vi "Lab Panel V5.31.vi"() -> ()   [LabVIEW 2017] (continued)
                        n3241 = Unbundle By Name(w5920) -> ("1 (TL) cal"=w5915:dbl, "1 (TN) cal"=w5914:dbl, "2 (TL) cal"=w5913:dbl, "2 (TN) cal"=w5912:dbl)  [unwired: 6 out]
                        n3242 = local write "TEMP LA03"(w5909) -> ()
                        n3243 = Multiply(x=w5908, y=w5915) -> (x*y=w5901:dbl)
                        n3244 = Multiply(x=w5907, y=w5914) -> (x*y=w5900:dbl)
                        n3245 = Multiply(x=w5906, y=w5913) -> (x*y=w5897:dbl)
                        n3246 = Multiply(x=w5905, y=w5912) -> (x*y=w5896:dbl)
                        n3247 = case shown="True" w5892 {
                          tunnel: w5897 -> [w5922 w5927]
                          tunnel: w5902 -> [_ w5925]
                          tunnel: [w5922 w5926] -> w5895
                          tunnel: w5896 -> [w5921 w5924]
                          tunnel: [w5921 w5923] -> w5894
                          frame False {
                          }
                          frame True {
                            n3248 = Multiply(x=w5925, y=w5924) -> (x*y=w5923:dbl)
                            n3249 = Multiply(x=w5925, y=w5927) -> (x*y=w5926:dbl)
                          }
                        }
                        n3250 = case shown="True" w5893 {
                          tunnel: w5901 -> [w5929 w5934]
                          tunnel: w5902 -> [_ w5932]
                          tunnel: [w5929 w5933] -> w5899
                          tunnel: w5900 -> [w5928 w5931]
                          tunnel: [w5928 w5930] -> w5898
                          frame False {
                          }
                          frame True {
                            n3251 = Multiply(x=w5932, y=w5931) -> (x*y=w5930:dbl)
                            n3252 = Multiply(x=w5932, y=w5934) -> (x*y=w5933:dbl)
                          }
                        }
                        n3253 = local read "SIG LAB03-2"() -> (w5917:T2)
                        n3254 = local read "SIG LAB03-1"() -> (w5919:T2)
                        n3255 = Bundle By Name(cluster=w5917, "Tmp Live"=w5895, "Tmp Neut"=w5894) -> (w5916:T2)
                        n3256 = Bundle By Name(cluster=w5919, "Tmp Live"=w5899, "Tmp Neut"=w5898) -> (w5918:T2)
                        n3257 = local write "SIG LAB03-2"(w5916) -> ()
                        n3258 = local write "SIG LAB03-1"(w5918) -> ()
                      }
                      frame #4 {
                        n3259 = case shown="False" w5949 {
                          tunnel: [w5980 w5981] -> w5965
                          tunnel: w5948 -> [_ w5981]
                          frame False {
                            n3260 = local read "CAL LAB04"() -> (w5980:T15)
                          }
                          frame True {
                          }
                        }
                        n3261 = local read "LAB04 TEMP"() -> (w5955:T13)
                        n3262 = local read "TEMP LA04"() -> (w5956:T10)
                        n3263 = call "sub vi - temperature delay v4.vi"("2-run"=w5937, "1-run"=w5938, "temp values IN"=w5956, "temp signals"=w5955) -> ("T2-N"=w5950:dbl, "T2-L"=w5951:dbl, "T1-N"=w5952:dbl, "T1-L"=w5953:dbl, "temp values OUT"=w5954:T47)  [unwired: 3 in]
                        n3264 = Unbundle By Name(w5965) -> ("1 (TL) cal"=w5960:dbl, "1 (TN) cal"=w5959:dbl, "2 (TL) cal"=w5958:dbl, "2 (TN) cal"=w5957:dbl)  [unwired: 6 out]
                        n3265 = local write "TEMP LA04"(w5954) -> ()
                        n3266 = Multiply(x=w5953, y=w5960) -> (x*y=w5946:dbl)
                        n3267 = Multiply(x=w5952, y=w5959) -> (x*y=w5945:dbl)
                        n3268 = Multiply(x=w5951, y=w5958) -> (x*y=w5942:dbl)
                        n3269 = Multiply(x=w5950, y=w5957) -> (x*y=w5941:dbl)
                        n3270 = case shown="True" w5937 {
                          tunnel: w5942 -> [w5967 w5972]
                          tunnel: w5947 -> [_ w5970]
                          tunnel: [w5967 w5971] -> w5940
                          tunnel: w5941 -> [w5966 w5969]
                          tunnel: [w5966 w5968] -> w5939
                          frame False {
                          }
                          frame True {
                            n3271 = Multiply(x=w5970, y=w5969) -> (x*y=w5968:dbl)
                            n3272 = Multiply(x=w5970, y=w5972) -> (x*y=w5971:dbl)
                          }
                        }
                        n3273 = case shown="True" w5938 {
                          tunnel: w5946 -> [w5974 w5979]
                          tunnel: w5947 -> [_ w5977]
                          tunnel: [w5974 w5978] -> w5944
                          tunnel: w5945 -> [w5973 w5976]
                          tunnel: [w5973 w5975] -> w5943
                          frame False {
                          }
                          frame True {
                            n3274 = Multiply(x=w5977, y=w5976) -> (x*y=w5975:dbl)
                            n3275 = Multiply(x=w5977, y=w5979) -> (x*y=w5978:dbl)
                          }
                        }
                        n3276 = local read "SIG LAB04-2"() -> (w5962:T2)
                        n3277 = local read "SIG LAB04-1"() -> (w5964:T2)
                        n3278 = Bundle By Name(cluster=w5962, "Tmp Live"=w5940, "Tmp Neut"=w5939) -> (w5961:T2)
                        n3279 = Bundle By Name(cluster=w5964, "Tmp Live"=w5944, "Tmp Neut"=w5943) -> (w5963:T2)
                        n3280 = local write "SIG LAB04-2"(w5961) -> ()
                        n3281 = local write "SIG LAB04-1"(w5963) -> ()
                      }
                      frame #5 {
                        n3282 = case shown="False" w5994 {
                          tunnel: [w6025 w6026] -> w6010
                          tunnel: w5993 -> [_ w6026]
                          frame False {
                            n3283 = local read "CAL LAB05"() -> (w6025:T15)
                          }
                          frame True {
                          }
                        }
                        n3284 = local read "LAB05 TEMP"() -> (w6000:T13)
                        n3285 = local read "TEMP LA05"() -> (w6001:T10)
                        n3286 = call "sub vi - temperature delay v4.vi"("2-run"=w5982, "1-run"=w5983, "temp values IN"=w6001, "temp signals"=w6000) -> ("T2-N"=w5996:dbl, "T2-L"=w5997:dbl, "T1-N"=w5998:dbl, "T1-L"=w5999:dbl, "temp values OUT"=w5995:T47)  [unwired: 3 in]
                        n3287 = local write "TEMP LA05"(w5995) -> ()
                        n3288 = Unbundle By Name(w6010) -> ("1 (TL) cal"=w6002:dbl, "1 (TN) cal"=w6005:dbl, "2 (TL) cal"=w6004:dbl, "2 (TN) cal"=w6003:dbl)  [unwired: 6 out]
                        n3289 = Multiply(x=w5999, y=w6002) -> (x*y=w5991:dbl)
                        n3290 = Multiply(x=w5998, y=w6005) -> (x*y=w5990:dbl)
                        n3291 = Multiply(x=w5997, y=w6004) -> (x*y=w5987:dbl)
                        n3292 = Multiply(x=w5996, y=w6003) -> (x*y=w5986:dbl)
                        n3293 = case shown="True" w5982 {
                          tunnel: w5987 -> [w6012 w6017]
                          tunnel: w5992 -> [_ w6015]
                          tunnel: [w6012 w6016] -> w5985
                          tunnel: w5986 -> [w6011 w6014]
                          tunnel: [w6011 w6013] -> w5984
                          frame False {
                          }
                          frame True {
                            n3294 = Multiply(x=w6015, y=w6014) -> (x*y=w6013:dbl)
                            n3295 = Multiply(x=w6015, y=w6017) -> (x*y=w6016:dbl)
                          }
                        }
                        n3296 = case shown="True" w5983 {
                          tunnel: w5991 -> [w6019 w6024]
                          tunnel: w5992 -> [_ w6022]
                          tunnel: [w6019 w6023] -> w5989
                          tunnel: w5990 -> [w6018 w6021]
                          tunnel: [w6018 w6020] -> w5988
                          frame False {
                          }
                          frame True {
                            n3297 = Multiply(x=w6022, y=w6021) -> (x*y=w6020:dbl)
                            n3298 = Multiply(x=w6022, y=w6024) -> (x*y=w6023:dbl)
                          }
                        }
                        n3299 = local read "SIG LAB05-1"() -> (w6009:T2)
                        n3300 = Bundle By Name(cluster=w6009, "Tmp Live"=w5989, "Tmp Neut"=w5988) -> (w6008:T2)
                        n3301 = local read "SIG LAB05-2"() -> (w6007:T2)
                        n3302 = Bundle By Name(cluster=w6007, "Tmp Live"=w5985, "Tmp Neut"=w5984) -> (w6006:T2)
                        n3303 = local write "SIG LAB05-1"(w6008) -> ()
                        n3304 = local write "SIG LAB05-2"(w6006) -> ()
                      }
                      frame #6 {
                        w6127 = 150.0
                        # "check for thermocouple error, output >150 deg??"
                        n3305 = local read "SIG LAB01-2"() -> (w6136:T2)
                        n3306 = local read "SIG LAB01-1"() -> (w6137:T2)
                        n3307 = local read "SIG LAB04-1"() -> (w6130:T2)
                        n3308 = local read "SIG LAB04-2"() -> (w6131:T2)
                        n3309 = Unbundle By Name(w6137) -> ("Tmp Live"=w6065:dbl, "Tmp Neut"=w6063:dbl)
                        n3310 = Unbundle(w6131) -> ("Tmp Live"=w6041:dbl, "Tmp Neut"=w6040:dbl)  [unwired: 3 out]
                        n3311 = Unbundle(w6136) -> ("Tmp Live"=w6062:dbl, "Tmp Neut"=w6060:dbl)  [unwired: 3 out]
                        n3312 = Unbundle(w6130) -> ("Tmp Live"=w6042:dbl, "Tmp Neut"=w6035:dbl)  [unwired: 3 out]
                        n3313 = Absolute Value(x=w6042) -> (abs(x)=w6036:dbl)
                        n3314 = Absolute Value(x=w6035) -> (abs(x)=w6037:dbl)
                        n3315 = Absolute Value(x=w6041) -> (abs(x)=w6039:dbl)
                        n3316 = Absolute Value(x=w6040) -> (abs(x)=w6038:dbl)
                        n3317 = Absolute Value(x=w6062) -> (abs(x)=w6061:dbl)
                        n3318 = Absolute Value(x=w6060) -> (abs(x)=w6059:dbl)
                        n3319 = Absolute Value(x=w6063) -> (abs(x)=w6064:dbl)
                        n3320 = Absolute Value(x=w6065) -> (abs(x)=w6066:dbl)
                        n3321 = Greater?(x=w6038, y=w6127) -> (0:w6103:bool)
                        "LA04-2 (TN)" <- w6103
                        n3322 = Greater?(x=w6059, y=w6127) -> (0:w6115:bool)
                        "LA01-2 (TN)" <- w6115
                        n3323 = Greater?(x=w6039, y=w6127) -> (0:w6104:bool)
                        "LA04-2 (TL)" <- w6104
                        n3324 = Greater?(x=w6061, y=w6127) -> (0:w6116:bool)
                        "LA01-2 (TL)" <- w6116
                        n3325 = Greater?(x=w6037, y=w6127) -> (0:w6105:bool)
                        "LA04-1 (TN)" <- w6105
                        n3326 = Greater?(x=w6064, y=w6127) -> (0:w6126:bool)
                        "LA01-1 (TN)" <- w6126
                        n3327 = Greater?(x=w6036, y=w6127) -> (0:w6106:bool)
                        "LA04-1 (TL)" <- w6106
                        n3328 = Greater?(x=w6066, y=w6127) -> (0:w6125:bool)
                        "LA01-1 (TL)" <- w6125
                        n3329 = Or(x=w6126, y=w6125) -> (x .or. y?=w6124:bool)
                        n3330 = Or(x=w6103, y=w6104) -> (x .or. y?=w6114:bool)
                        n3331 = Or(x=w6116, y=w6115) -> (x .or. y?=w6120:bool)
                        n3332 = Or(x=w6105, y=w6106) -> (x .or. y?=w6110:bool)
                        n3333 = Select(t=u32 16711680, s=w6124, f=u32 13816530) -> (s? t:f=w6121:u32)
                        n3334 = Select(t=u32 16711680, s=w6114, f=u32 13816530) -> (s? t:f=w6111:u32)
                        n3335 = Select(t=u32 16711680, s=w6120, f=u32 13816530) -> (s? t:f=w6117:u32)
                        n3336 = Select(t=u32 16711680, s=w6110, f=u32 13816530) -> (s? t:f=w6107:u32)
                        n3337 = property on="SIG LAB01-1" class="Clust (strict)"("Color"=w6121) -> ()  [unwired: 2 in, 2 out]
                        n3338 = property on="SIG LAB01-2" class="Clust (strict)"("Color"=w6117) -> ()  [unwired: 2 in, 2 out]
                        n3339 = property on="SIG LAB04-2" class="Clust (strict)"("Color"=w6111) -> ()  [unwired: 2 in, 2 out]
                        n3340 = property on="SIG LAB04-1" class="Clust (strict)"("Color"=w6107) -> ()  [unwired: 2 in, 2 out]
                        n3341 = local read "SIG LAB02-1"() -> (w6134:T2)
                        n3342 = local read "SIG LAB02-2"() -> (w6135:T2)
                        n3343 = local read "SIG LAB05-2"() -> (w6128:T2)
                        n3344 = local read "SIG LAB05-1"() -> (w6129:T2)
                        n3345 = Unbundle(w6135) -> ("Tmp Live"=w6054:dbl, "Tmp Neut"=w6052:dbl)  [unwired: 3 out]
                        n3346 = Unbundle(w6134) -> ("Tmp Live"=w6058:dbl, "Tmp Neut"=w6057:dbl)  [unwired: 3 out]
                        n3347 = Unbundle(w6128) -> ("Tmp Live"=w6030:dbl, "Tmp Neut"=w6028:dbl)  [unwired: 3 out]
                        n3348 = Unbundle(w6129) -> ("Tmp Live"=w6034:dbl, "Tmp Neut"=w6032:dbl)  [unwired: 3 out]
                        n3349 = Absolute Value(x=w6054) -> (abs(x)=w6053:dbl)
                        n3350 = Absolute Value(x=w6052) -> (abs(x)=w6051:dbl)
                        n3351 = Absolute Value(x=w6057) -> (abs(x)=w6055:dbl)
                        n3352 = Absolute Value(x=w6058) -> (abs(x)=w6056:dbl)
                        n3353 = Absolute Value(x=w6030) -> (abs(x)=w6029:dbl)
                        n3354 = Absolute Value(x=w6028) -> (abs(x)=w6027:dbl)
                        n3355 = Absolute Value(x=w6034) -> (abs(x)=w6033:dbl)
                        n3356 = Absolute Value(x=w6032) -> (abs(x)=w6031:dbl)
                        n3357 = Greater?(x=w6051, y=w6127) -> (0:w6079:bool)
                        "LA02-2 (TN)" <- w6079
                        n3358 = Greater?(x=w6053, y=w6127) -> (0:w6080:bool)
                        "LA02-2 (TL)" <- w6080
                        n3359 = Greater?(x=w6055, y=w6127) -> (0:w6082:bool)
                        "LA02-1 (TN)" <- w6082
                        n3360 = Greater?(x=w6056, y=w6127) -> (0:w6081:bool)
                        "LA02-1 (TL)" <- w6081
                        n3361 = Greater?(x=w6027, y=w6127) -> (0:w6091:bool)
                        "LA05-2 (TN)" <- w6091
                        n3362 = Greater?(x=w6029, y=w6127) -> (0:w6092:bool)
                        "LA05-2 (TL)" <- w6092
                        n3363 = Greater?(x=w6031, y=w6127) -> (0:w6093:bool)
                        "LA05-1 (TN)" <- w6093
                        n3364 = Greater?(x=w6033, y=w6127) -> (0:w6094:bool)
                        "LA05-1 (TL)" <- w6094
                        n3365 = Or(x=w6082, y=w6081) -> (x .or. y?=w6090:bool)
                        n3366 = Or(x=w6080, y=w6079) -> (x .or. y?=w6086:bool)
                        n3367 = Or(x=w6094, y=w6093) -> (x .or. y?=w6102:bool)
                        n3368 = Or(x=w6092, y=w6091) -> (x .or. y?=w6098:bool)
                        n3369 = Select(t=u32 16711680, s=w6090, f=u32 13816530) -> (s? t:f=w6087:u32)
                        n3370 = Select(t=u32 16711680, s=w6086, f=u32 13816530) -> (s? t:f=w6083:u32)
                        n3371 = Select(t=u32 16711680, s=w6102, f=u32 13816530) -> (s? t:f=w6099:u32)
                        n3372 = local read "SIG LAB03-1"() -> (w6132:T2)
                        n3373 = Select(t=u32 16711680, s=w6098, f=u32 13816530) -> (s? t:f=w6095:u32)
                        n3374 = property on="SIG LAB02-1" class="Clust (strict)"("Color"=w6087) -> ()  [unwired: 2 in, 2 out]
                        n3375 = property on="SIG LAB02-2" class="Clust (strict)"("Color"=w6083) -> ()  [unwired: 2 in, 2 out]
                        n3376 = local read "SIG LAB03-2"() -> (w6133:T2)
                        n3377 = property on="SIG LAB05-1" class="Clust (strict)"("Color"=w6099) -> ()  [unwired: 2 in, 2 out]
                        n3378 = property on="SIG LAB05-2" class="Clust (strict)"("Color"=w6095) -> ()  [unwired: 2 in, 2 out]
                        n3379 = Unbundle(w6133) -> ("Tmp Live"=w6046:dbl, "Tmp Neut"=w6044:dbl)  [unwired: 3 out]
                        n3380 = Unbundle(w6132) -> ("Tmp Live"=w6050:dbl, "Tmp Neut"=w6048:dbl)  [unwired: 3 out]
                        n3381 = Absolute Value(x=w6046) -> (abs(x)=w6045:dbl)
                        n3382 = Absolute Value(x=w6044) -> (abs(x)=w6043:dbl)
                        n3383 = Absolute Value(x=w6050) -> (abs(x)=w6049:dbl)
                        n3384 = Absolute Value(x=w6048) -> (abs(x)=w6047:dbl)
                        n3385 = Greater?(x=w6043, y=w6127) -> (0:w6067:bool)
                        "LA03-2 (TN)" <- w6067
                        n3386 = Greater?(x=w6045, y=w6127) -> (0:w6068:bool)
                        "LA03-2 (TL)" <- w6068
                        n3387 = Greater?(x=w6047, y=w6127) -> (0:w6070:bool)
                        "LA03-1 (TN)" <- w6070
                        n3388 = Greater?(x=w6049, y=w6127) -> (0:w6069:bool)
                        "LA03-1 (TL)" <- w6069
                        n3389 = Or(x=w6070, y=w6069) -> (x .or. y?=w6078:bool)
                        n3390 = Or(x=w6068, y=w6067) -> (x .or. y?=w6074:bool)
                        n3391 = Select(t=u32 16711680, s=w6078, f=u32 13816530) -> (s? t:f=w6075:u32)
                        n3392 = Select(t=u32 16711680, s=w6074, f=u32 13816530) -> (s? t:f=w6071:u32)
                        n3393 = property on="SIG LAB03-1" class="Clust (strict)"("Color"=w6075) -> ()  [unwired: 2 in, 2 out]
                        n3394 = property on="SIG LAB03-2" class="Clust (strict)"("Color"=w6071) -> ()  [unwired: 2 in, 2 out]
                      }
                    }
                  }
                }
              }
            }
          }
          frame #22 {
            # "SAVE ON AMPS VALUES FOR REPORT FILE"
            # "write data to display panel"
            n3395 = global write "Global display 1.vi" "TEST 5-2"(w6173) -> ()
            n3396 = global write "Global display 1.vi" "TEST 4-2"(w6175) -> ()
            n3397 = global write "Global display 1.vi" "TEST 1-2"(w6181) -> ()
            n3398 = global write "Global display 1.vi" "TEST 3-1"(w6178) -> ()
            n3399 = global write "Global display 1.vi" "TEST 5-1"(w6174) -> ()
            n3400 = global write "Global display 1.vi" "TEST 1-1"(w6182) -> ()
            n3401 = global write "Global display 1.vi" "TEST 3-2"(w6177) -> ()
            n3402 = global write "Global display 1.vi" "TEST 4-1"(w6176) -> ()
            n3403 = global write "Global display 1.vi" "TEST 2-2"(w6179) -> ()
            n3404 = global write "Global display 1.vi" "TEST 2-1"(w6180) -> ()
            n3405 = global read "Global display 3.vi" "log 1-1"() -> (→"LOG LAB01-1":string)
            n3406 = global read "Global display 3.vi" "log 3-1"() -> (→"LOG LAB03-1":string)
            n3407 = global read "Global display 3.vi" "log 1-2"() -> (→"LOG LAB01-2":string)
            n3408 = property on="Tab Control 2" class="TabCtl (strict)"() -> ("Pages"=w6172:refnum<vi>[])  [unwired: 2 in, 2 out]
            n3409 = global read "Global display 3.vi" "log 2-1"() -> (→"LOG LAB02-1":string)
            n3410 = global read "Global display 3.vi" "log 2-2"() -> (→"LOG LAB02-2":string)
            n3411 = global read "Global display 3.vi" "log 4-2"() -> (→"LOG LAB04-2":string)
            n3412 = global read "Global display 3.vi" "log 5-2"() -> (→"LOG LAB05-2":string)
            n3413 = global read "Global display 3.vi" "log 5-1"() -> (→"LOG LAB05-1":string)
            n3414 = global read "Global display 3.vi" "log 4-1"() -> (→"LOG LAB04-1":string)
            n3415 = global read "Global display 3.vi" "log 3-2"() -> (→"LOG LAB03-2":string)
            n3416 = Index Array(array=w6172, index=8) -> (element=w6170:refnum<vi>)
            n3417 = property class="Page"(reference=w6170) -> ("PageVis"=w6169:bool)  [unwired: 1 in, 2 out]
            n3418 = local read "DISP LAB03-1"() -> (w6208:T4)
            n3419 = local read "DISP LAB04-2"() -> (w6205:T4)
            n3420 = local read "DISP LAB05-1"() -> (w6204:T4)
            n3421 = local read "DISP LAB01-2"() -> (w6211:T4)
            n3422 = local read "DISP LAB02-1"() -> (w6210:T4)
            n3423 = local read "DISP LAB02-2"() -> (w6209:T4)
            n3424 = local read "DISP LAB04-1"() -> (w6206:T4)
            n3425 = local read "DISP LAB05-2"() -> (w6203:T4)
            n3426 = local read "DISP LAB01-1"() -> (w6212:T4)
            n3427 = local read "DISP LAB03-2"() -> (w6207:T4)
            n3428 = global write "Global display 3.vi" "admin"(w6169) -> ()
            n3429 = local read "O/I  LAB05-2"() -> (w6223:bool)
            n3430 = local read "O/I  LAB05-1"() -> (w6224:bool)
            n3431 = local read "O/I  LAB03-2"() -> (w6227:bool)
            n3432 = local read "O/I  LAB04-2"() -> (w6225:bool)
            n3433 = local read "O/I  LAB04-1"() -> (w6226:bool)
            n3434 = local read "O/I  LAB03-1"() -> (w6228:bool)
            n3435 = local read "O/I  LAB01-2"() -> (w6231:bool)
            n3436 = local read "O/I  LAB01-1"() -> (w6232:bool)
            n3437 = local read "O/I  LAB02-1"() -> (w6230:bool)
            n3438 = local read "O/I  LAB02-2"() -> (w6229:bool)
            n3439 = global write "Global display 1.vi" "5-2 O/F"(w6223) -> ()
            n3440 = global write "Global display 1.vi" "5-1 O/F"(w6224) -> ()
            n3441 = global write "Global display 1.vi" "4-1 O/F"(w6226) -> ()
            n3442 = global write "Global display 1.vi" "4-2 O/F"(w6225) -> ()
            n3443 = global write "Global display 2.vi" "DISP LAB02-1"(w6210) -> ()
            n3444 = global write "Global display 2.vi" "DISP LAB02-2"(w6209) -> ()
            n3445 = global write "Global display 2.vi" "DISP LAB05-1"(w6204) -> ()
            n3446 = global write "Global display 2.vi" "DISP LAB05-2"(w6203) -> ()
            n3447 = global write "Global display 1.vi" "3-2 O/F"(w6227) -> ()
            n3448 = global write "Global display 2.vi" "DISP LAB01-2"(w6211) -> ()
            n3449 = global write "Global display 2.vi" "DISP LAB04-2"(w6205) -> ()
            n3450 = global write "Global display 2.vi" "DISP LAB01-1"(w6212) -> ()
            n3451 = global write "Global display 2.vi" "DISP LAB03-1"(w6208) -> ()
            n3452 = global write "Global display 1.vi" "3-1 O/F"(w6228) -> ()
            n3453 = global write "Global display 2.vi" "DISP LAB04-1"(w6206) -> ()
            n3454 = global write "Global display 1.vi" "2-2 O/F"(w6229) -> ()
            n3455 = global write "Global display 2.vi" "DISP LAB03-2"(w6207) -> ()
            n3456 = global write "Global display 1.vi" "2-1 O/F"(w6230) -> ()
            n3457 = global write "Global display 1.vi" "1-2 O/F"(w6231) -> ()
            n3458 = global write "Global display 1.vi" "1-1 O/F"(w6232) -> ()
            n3459 = local read "run lab05-2"() -> (w6213:bool)
            n3460 = local read "run lab04-1"() -> (w6216:bool)
            n3461 = local read "run lab04-2"() -> (w6215:bool)
            n3462 = local read "run lab05-1"() -> (w6214:bool)
            n3463 = local read "TEMP START LAB02-2"() -> (w6155:cluster{"TL":dbl, "TN":dbl})
            n3464 = local read "TEMP START LAB01-2"() -> (w6157:cluster{"TL":dbl, "TN":dbl})
            n3465 = local read "TEMP START LAB02-1"() -> (w6156:cluster{"TL":dbl, "TN":dbl})
            n3466 = local read "TEMP START LAB04-1"() -> (w6152:cluster{"TL":dbl, "TN":dbl})
            n3467 = local read "TEMP START LAB04-2"() -> (w6151:cluster{"TL":dbl, "TN":dbl})
            n3468 = local read "run lab03-2"() -> (w6217:bool)
            n3469 = local read "TEMP START LAB01-1"() -> (w6158:cluster{"TL":dbl, "TN":dbl})
            n3470 = local read "TEMP START LAB05-2"() -> (w6149:cluster{"TL":dbl, "TN":dbl})
            n3471 = local read "TEMP START LAB05-1"() -> (w6150:cluster{"TL":dbl, "TN":dbl})
            n3472 = local read "run lab02-1"() -> (w6220:bool)
            n3473 = local read "run lab03-1"() -> (w6218:bool)
            n3474 = local read "TEMP START LAB03-2"() -> (w6153:cluster{"TL":dbl, "TN":dbl})
            n3475 = local read "run lab01-2"() -> (w6221:bool)
            n3476 = local read "run lab02-2"() -> (w6219:bool)
            n3477 = local read "TEMP START LAB03-1"() -> (w6154:cluster{"TL":dbl, "TN":dbl})
            n3478 = local read "run lab01-1"() -> (w6222:bool)
            n3479 = global write "Global display 1.vi" "5-2 R/S"(w6213) -> ()
            n3480 = global write "Global display 1.vi" "5-1 R/S"(w6214) -> ()
            n3481 = global write "Global display 1.vi" "4-2 R/S"(w6215) -> ()
            n3482 = global write "Global display 1.vi" "4-1 R/S"(w6216) -> ()
            n3483 = global write "Global display 1.vi" "3-2 R/S"(w6217) -> ()
            n3484 = global write "Global display 1.vi" "1-2 R/S"(w6221) -> ()
            n3485 = global write "Global display 1.vi" "2-1 R/S"(w6220) -> ()
            n3486 = global write "Global display 1.vi" "3-1 R/S"(w6218) -> ()
            n3487 = global write "Global display 1.vi" "2-2 R/S"(w6219) -> ()
            n3488 = global write "Global display 1.vi" "1-1 R/S"(w6222) -> ()
            n3489 = local read "SET LAB05-2"() -> (w6193:T5)
            n3490 = local read "SET LAB05-1"() -> (w6194:T5)
            n3491 = local read "SET LAB04-1"() -> (w6196:T5)
            n3492 = local read "SET LAB04-2"() -> (w6195:T5)
            n3493 = local read "SET LAB01-1"() -> (w6202:T6)
            n3494 = local read "SET LAB03-1"() -> (w6198:T5)
            n3495 = local read "SET LAB03-2"() -> (w6197:T5)
            n3496 = local read "SET LAB02-2"() -> (w6199:T5)
            n3497 = local read "SET LAB01-2"() -> (w6201:T5)
            n3498 = local read "SET LAB02-1"() -> (w6200:T5)
            n3499 = global write "Global display 3.vi" "TEMP ST 05-2"(w6149) -> ()
            n3500 = global write "Global display 3.vi" "TEMP ST 05-1"(w6150) -> ()
            n3501 = global write "Global display 3.vi" "TEMP ST 03-2"(w6153) -> ()
            n3502 = global write "Global display 3.vi" "TEMP ST 04-2"(w6151) -> ()
            n3503 = global write "Global display 3.vi" "TEMP ST 01-1"(w6158) -> ()
            n3504 = global write "Global display 3.vi" "TEMP ST 01-2"(w6157) -> ()
            n3505 = global write "Global display 3.vi" "TEMP ST 04-1"(w6152) -> ()
            n3506 = global write "Global display 3.vi" "TEMP ST 02-1"(w6156) -> ()
            n3507 = global write "Global display 3.vi" "TEMP ST 02-2"(w6155) -> ()
            n3508 = global write "Global display 3.vi" "TEMP ST 03-1"(w6154) -> ()
            n3509 = global write "Global display 2.vi" "SET LAB05-2"(w6193) -> ()
            n3510 = global write "Global display 2.vi" "SET LAB05-1"(w6194) -> ()
            n3511 = global write "Global display 2.vi" "SET LAB04-1"(w6196) -> ()
            n3512 = global write "Global display 2.vi" "SET LAB01-1"(w6202) -> ()
            n3513 = global write "Global display 2.vi" "SET LAB04-2"(w6195) -> ()
            n3514 = global write "Global display 2.vi" "SET LAB03-2"(w6197) -> ()
            n3515 = global write "Global display 2.vi" "SET LAB02-2"(w6199) -> ()
            n3516 = global write "Global display 2.vi" "SET LAB03-1"(w6198) -> ()
            n3517 = global write "Global display 2.vi" "SET LAB01-2"(w6201) -> ()
            n3518 = global write "Global display 2.vi" "SET LAB02-1"(w6200) -> ()
            n3519 = local read "TEMP RISE LAB05-1"() -> (w6140:cluster{"TL":dbl, "TN":dbl})
            n3520 = local read "TEMP RISE LAB05-2"() -> (w6139:cluster{"TL":dbl, "TN":dbl})
            n3521 = local read "TEMP RISE LAB04-2"() -> (w6141:cluster{"TL":dbl, "TN":dbl})
            n3522 = local read "TEMP RISE LAB04-1"() -> (w6142:cluster{"TL":dbl, "TN":dbl})
            n3523 = local read "TEMP RISE LAB03-2"() -> (w6143:cluster{"TL":dbl, "TN":dbl})
            n3524 = local read "TEMP RISE LAB03-1"() -> (w6144:cluster{"TL":dbl, "TN":dbl})
            n3525 = local read "TEMP RISE LAB01-2"() -> (w6147:cluster{"TL":dbl, "TN":dbl})
            n3526 = local read "TEMP RISE LAB02-2"() -> (w6145:cluster{"TL":dbl, "TN":dbl})
            n3527 = local read "TEMP RISE LAB01-1"() -> (w6148:cluster{"TL":dbl, "TN":dbl})
            n3528 = local read "TEMP RISE LAB02-1"() -> (w6146:cluster{"TL":dbl, "TN":dbl})
            n3529 = local read "RESULT LAB01-1"() -> (w6192:bool)
            n3530 = local read "RESULT LAB03-2"() -> (w6187:bool)
            n3531 = local read "RESULT LAB04-1"() -> (w6186:bool)
            n3532 = local read "RESULT LAB04-2"() -> (w6185:bool)
            n3533 = local read "RESULT LAB02-2"() -> (w6189:bool)
            n3534 = local read "RESULT LAB01-2"() -> (w6191:bool)
            n3535 = local read "RESULT LAB02-1"() -> (w6190:bool)
            n3536 = local read "RESULT LAB03-1"() -> (w6188:bool)
            n3537 = local read "RESULT LAB05-1"() -> (w6184:bool)
            n3538 = local read "RESULT LAB05-2"() -> (w6183:bool)
            n3539 = local read "Amps Fail level"() -> (w6138:dbl)
            n3540 = stacked-sequence {
              tunnel: w6138 -> [w6234 w6239 w6244 w6249 w6254 w6259 w6264 w6269 w6274 w6279]
              frame #0 {
                n3541 = local read "SIG LAB01-1"() -> (w6236:T2)
                n3542 = Unbundle(w6236) -> ("AMPS"=w6235:dbl)  [unwired: 4 out]
                n3543 = Greater?(x=w6235, y=w6234) -> (0:w6233:bool)
                n3544 = case shown="True" w6233 {
                  frame False {
                  }
                  frame True {
                    n3545 = local read "ON L01-1"() -> (w6237:cluster{"amps":dbl, "volts":dbl, "pf":dbl})
                    n3546 = global write "Global display 2.vi" "ON L01-1"(w6237) -> ()
                  }
                }
              }
              frame #1 {
                n3547 = local read "SIG LAB01-2"() -> (w6241:T2)
                n3548 = Unbundle By Name(w6241) -> ("AMPS"=w6240:dbl)
                n3549 = Greater?(x=w6240, y=w6239) -> (0:w6238:bool)
                n3550 = case shown="True" w6238 {
                  frame False {
                  }
                  frame True {
                    n3551 = local read "ON L01-2"() -> (w6242:cluster{"amps":dbl, "volts":dbl, "pf":dbl})
                    n3552 = global write "Global display 2.vi" "ON L01-2"(w6242) -> ()
                  }
                }
              }
              frame #2 {
                n3553 = local read "SIG LAB02-1"() -> (w6246:T2)
                n3554 = Unbundle(w6246) -> ("AMPS"=w6245:dbl)  [unwired: 4 out]
                n3555 = Greater?(x=w6245, y=w6244) -> (0:w6243:bool)
                n3556 = case shown="True" w6243 {
                  frame False {
                  }
                  frame True {
                    n3557 = local read "ON L02-1"() -> (w6247:cluster{"amps":dbl, "volts":dbl, "pf":dbl})
                    n3558 = global write "Global display 2.vi" "ON L02-1"(w6247) -> ()
                  }
                }
              }
              frame #3 {
                n3559 = local read "SIG LAB02-2"() -> (w6251:T2)
                n3560 = Unbundle(w6251) -> ("AMPS"=w6250:dbl)  [unwired: 4 out]
                n3561 = Greater?(x=w6250, y=w6249) -> (0:w6248:bool)
                n3562 = case shown="True" w6248 {
                  frame False {
                  }
                  frame True {
                    n3563 = local read "ON L02-2"() -> (w6252:cluster{"amps":dbl, "volts":dbl, "pf":dbl})
                    n3564 = global write "Global display 2.vi" "ON L02-2"(w6252) -> ()
                  }
                }
              }
              frame #4 {
                n3565 = local read "SIG LAB03-1"() -> (w6256:T2)
                n3566 = Unbundle(w6256) -> ("AMPS"=w6255:dbl)  [unwired: 4 out]
                n3567 = Greater?(x=w6255, y=w6254) -> (0:w6253:bool)
                n3568 = case shown="True" w6253 {
                  frame False {
                  }
                  frame True {
                    n3569 = local read "ON L03-1"() -> (w6257:cluster{"amps":dbl, "volts":dbl, "pf":dbl})
                    n3570 = global write "Global display 2.vi" "ON L03-1"(w6257) -> ()
                  }
                }
              }
              frame #5 {
                n3571 = local read "SIG LAB03-2"() -> (w6261:T2)
                n3572 = Unbundle(w6261) -> ("AMPS"=w6260:dbl)  [unwired: 4 out]
                n3573 = Greater?(x=w6260, y=w6259) -> (0:w6258:bool)
                n3574 = case shown="True" w6258 {
                  frame False {
                  }
                  frame True {
                    n3575 = local read "ON L03-2"() -> (w6262:cluster{"amps":dbl, "volts":dbl, "pf":dbl})
                    n3576 = global write "Global display 2.vi" "ON L03-2"(w6262) -> ()
                  }
                }
              }
              frame #6 {
                n3577 = local read "SIG LAB04-1"() -> (w6266:T2)
                n3578 = Unbundle(w6266) -> ("AMPS"=w6265:dbl)  [unwired: 4 out]
                n3579 = Greater?(x=w6265, y=w6264) -> (0:w6263:bool)
                n3580 = case shown="True" w6263 {
                  frame False {
                  }
                  frame True {
                    n3581 = local read "ON L04-1"() -> (w6267:cluster{"amps":dbl, "volts":dbl, "pf":dbl})
                    n3582 = global write "Global display 2.vi" "ON L04-1"(w6267) -> ()
                  }
                }
              }
              frame #7 {
                n3583 = local read "SIG LAB04-2"() -> (w6271:T2)
                n3584 = Unbundle(w6271) -> ("AMPS"=w6270:dbl)  [unwired: 4 out]
                n3585 = Greater?(x=w6270, y=w6269) -> (0:w6268:bool)
                n3586 = case shown="True" w6268 {
                  frame False {
                  }
                  frame True {
                    n3587 = local read "ON L04-2"() -> (w6272:cluster{"amps":dbl, "volts":dbl, "pf":dbl})
                    n3588 = global write "Global display 2.vi" "ON L04-2"(w6272) -> ()
                  }
                }
              }
              frame #8 {
                n3589 = local read "SIG LAB05-1"() -> (w6276:T2)
                n3590 = Unbundle(w6276) -> ("AMPS"=w6275:dbl)  [unwired: 4 out]
                n3591 = Greater?(x=w6275, y=w6274) -> (0:w6273:bool)
                n3592 = case shown="True" w6273 {
                  frame False {
                  }
                  frame True {
                    n3593 = local read "ON L05-1"() -> (w6277:cluster{"amps":dbl, "volts":dbl, "pf":dbl})
                    n3594 = global write "Global display 2.vi" "ON L05-1"(w6277) -> ()
                  }
                }
              }
              frame #9 {
                n3595 = local read "SIG LAB05-2"() -> (w6281:T2)
                n3596 = Unbundle(w6281) -> ("AMPS"=w6280:dbl)  [unwired: 4 out]
                n3597 = Greater?(x=w6280, y=w6279) -> (0:w6278:bool)
                n3598 = case shown="True" w6278 {
                  frame False {
                  }
                  frame True {
                    n3599 = local read "ON L05-2"() -> (w6282:cluster{"amps":dbl, "volts":dbl, "pf":dbl})
                    n3600 = global write "Global display 2.vi" "ON L05-2"(w6282) -> ()
                  }
                }
              }
            }
            n3601 = global write "Global display 3.vi" "TEMP RS 05-2"(w6139) -> ()
            n3602 = global write "Global display 3.vi" "TEMP RS 05-1"(w6140) -> ()
            n3603 = global write "Global display 3.vi" "TEMP RS 03-2"(w6143) -> ()
            n3604 = global write "Global display 3.vi" "TEMP RS 02-1"(w6146) -> ()
            n3605 = global write "Global display 3.vi" "TEMP RS 02-2"(w6145) -> ()
            n3606 = global write "Global display 3.vi" "TEMP RS 04-2"(w6141) -> ()
            n3607 = global write "Global display 3.vi" "TEMP RS 01-2"(w6147) -> ()
            n3608 = global write "Global display 3.vi" "TEMP RS 03-1"(w6144) -> ()
            n3609 = global write "Global display 3.vi" "TEMP RS 04-1"(w6142) -> ()
            n3610 = global write "Global display 3.vi" "TEMP RS 01-1"(w6148) -> ()
            n3611 = global write "Global display 2.vi" "RESULT LAB05-1"(w6184) -> ()
            n3612 = global write "Global display 2.vi" "RESULT LAB01-2"(w6191) -> ()
            n3613 = global write "Global display 2.vi" "RESULT LAB03-2"(w6187) -> ()
            n3614 = global write "Global display 2.vi" "RESULT LAB04-1"(w6186) -> ()
            n3615 = global write "Global display 2.vi" "RESULT LAB04-2"(w6185) -> ()
            n3616 = global write "Global display 2.vi" "RESULT LAB05-2"(w6183) -> ()
            n3617 = global write "Global display 2.vi" "RESULT LAB03-1"(w6188) -> ()
            n3618 = global write "Global display 2.vi" "RESULT LAB01-1"(w6192) -> ()
            n3619 = global write "Global display 2.vi" "RESULT LAB02-1"(w6190) -> ()
            n3620 = global write "Global display 2.vi" "RESULT LAB02-2"(w6189) -> ()
          }
          frame #23 {
            # "simulate values"
            n3621 = global write "Global display 4.vi" "LAB deg C"("LAB deg C") -> ()
          }
          frame #24 {
            # "end main and display program"
            n3622 = stacked-sequence {
              seq-local: [_ w6289 _] -> [_ _ w6295]
              tunnel: w6285 -> [w6286 _ _]
              tunnel: w6284 -> [_ _ w6293]
              frame #0 {
                n3623 = case shown="True" w6286 {
                  frame False {
                  }
                  frame True {
                    n3624 = One Button Dialog(message="Excessive number of USB \nresets done, re-start program.") -> ()  [unwired: 1 in, 1 out]
                  }
                }
              }
              frame #1 {
                # "check for reset error"
                n3625 = local read "Simulate"() -> (w6288:bool)
                n3626 = case shown="False" w6288 {
                  tunnel: [w6290 FALSE] -> w6289
                  frame False {
                    n3627 = local read "Reset Error"() -> (w6290:bool)
                    n3628 = case shown="True" w6290 {
                      frame False {
                      }
                      frame True {
                        n3629 = One Button Dialog(message="USB ERROR, program will be stopped.\nClose program, close windows, switch panel off\nand re power panel. If error persists seek help.") -> ()  [unwired: 1 in, 1 out]
                      }
                    }
                  }
                  frame True {
                  }
                }
              }
              frame #2 {
                # "end labview session"
                n3630 = case shown="True" w6293 {
                  frame False {
                  }
                  frame True {
                    n3631 = call "sub vi - AI USB4704 (3)  Close Task v2.vi"() -> ()  [unwired: 16 in]
                  }
                }
                n3632 = Or(x=w6295, y="stop all") -> (x .or. y?=w6294:bool)
                n3633 = case shown="True" w6294 {
                  frame False {
                  }
                  frame True {
                    n3634 = stacked-sequence {
                      frame #0 {
                        n3635 = global write "Global display 1.vi" "stop disp"(TRUE) -> ()
                      }
                      frame #1 {
                        n3636 = call "sub vi - AI USB4704 (3)  Close Task v2.vi"() -> ()  [unwired: 16 in]
                      }
                      frame #2 {
                        n3637 = Quit LabVIEW(quit? (T)=TRUE) -> ()
                      }
                    }
                  }
                }
              }
            }
          }
        }
        n3638 = node-c288() -> ()  [unwired: 1 in, 1 out]
        "loops" <- w350
      }
      n3639 = node-c288(w322) -> ()  [unwired: 1 out]
    }
  }
